vi "TokenSort.vi"(10 "Token":string) -> (2 "TokenType":T1)   [LabVIEW 2009]
uses:
  TokenType.ctl
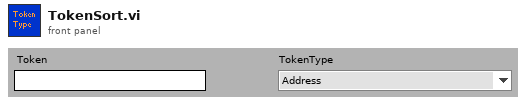
[diagram p1: front panel]
types:
  T1 = typedef "TokenType.ctl" = enum16{"Address", "TransID", "Content"}
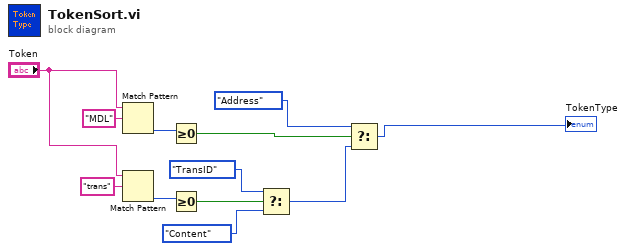
[diagram p0: block diagram]
diagram:
  n1 = Match Pattern(string="Token", regular expression="MDL") -> (offset past match=w11:i32)  [unwired: 4 out]
  n2 = Match Pattern(string="Token", regular expression="trans") -> (offset past match=w9:i32)  [unwired: 4 out]
  n3 = Greater Or Equal To 0?(x=w11) -> (x >= 0?=w7:bool)
  n4 = Greater Or Equal To 0?(x=w9) -> (x >= 0?=w6:bool)
  n5 = Select(t=TokenType."TransID" ("TokenType"), s=w6, f=TokenType."Content" ("TokenType")) -> (s? t:f=w5:T1)
  n6 = Select(t=TokenType."Address" ("TokenType"), s=w7, f=w5) -> (s? t:f=→"TokenType":T1)
